vi "Render Non-False Section.vi"(8 "Error In":errorcluster) -> (0 "Error Out":errorcluster)   [LabVIEW 2018, in "Tests.lvlib" / "Render.lvlib"]
uses:
  Render.lvlib
  <vilib>/addons/_JKI Toolkits/Caraya/classes/Test/Test.lvclass
  <vilib>/addons/_JKI Toolkits/Caraya/classes/Assert/Assert.lvclass
  src/Toolkit/Toolkit.lvlib
  src/Toolkit/Data/Map/Map.lvclass
  src/Toolkit/Low-Level/Support/Lex String.vi
  src/Toolkit/Low-Level/Support/Render to String.vi
  src/Toolkit/Data/Map/Support/From String.vi
  src/Toolkit/Low-Level/Context/Compiler.lvclass
  D:/Users/cfield/Code/Field R&D Services/Labstache/src/Toolkit/Data/Datum/Datum.lvclass
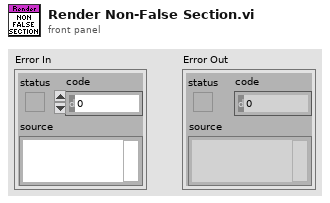
[diagram p1: front panel]
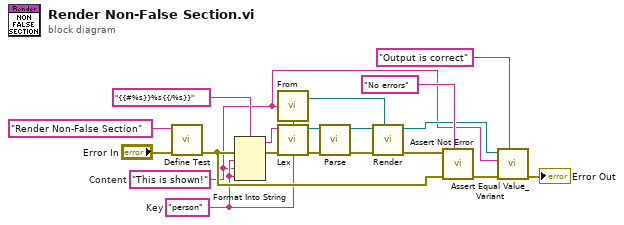
[diagram p0: block diagram]
diagram:
  w1 = "This is shown!"  # Content
  w3 = "person"  # Key
  n1 = call <vilib>:"Define Test.vi"("error in (no error)"="Error In", "Label (VI Title)"="Render Non-False Section") -> ("error out"=w7:errorcluster)  [unwired: 9 in]
  n2 = Format Into String(format string="{{#%s}}%s{{/%s}}", error in=w7, w3, w1, w3) -> (resulting string=w4:string, error out=w6:errorcluster)  [unwired: 1 in]
  n3 = call-poly "From.vi"("Value"=w1, "Key"=w3) -> ("Map"=w8:refnum<class "Map.lvclass">)
  n4 = call-poly "Lex.vi"("Error In"=w6, "Context In"=w4) -> ("Error Out"=w9:errorcluster, "Context Out"=w10:refnum<class "Compiler.lvclass">)  [unwired: 7 in, 1 out]
  n5 = call "Parse.vi"("Error In"=w9, "Context In"=w10) -> ("Error Out"=w11:errorcluster, "Context Out"=w2:refnum<class "Compiler.lvclass">)  [unwired: 7 in, 1 out]
  n6 = call-poly "Render.vi"(7:w8, "Error In"=w11, "Context In"=w2) -> ("Error Out"=w13:errorcluster, "Context Out"=w12:refnum<class "Compiler.lvclass">)  [unwired: 6 in, 1 out]
  n7 = call <vilib>:"Assert Not Error.vi"("Label"="No errors", "error in (no error)"=w7, "Not Error?"=w13) -> ("error out"=w16:errorcluster)  [unwired: 8 in]
  n8 = call <vilib>:"Assert Equal Value_Variant.vi"("Label"="Output is correct", "error in (no error)"=w16, "Y"=w1, "X"=w12) -> ("error out"=→"Error Out":errorcluster)  [unwired: 7 in]
